vi "SwerveDrivePoseEst2_Execute.vi"(0 "Vision TImeStamp_Seconds":dbl=0.02, 3 "DiffPoseEst2Config":T3={"Wheel_Locations M"=[], "Odom X std dev M"=0.02, "Odom Y std dev M"=0.02, "Odom Heading std dev Rad"=0.01, "Vision X std dev M"=0.1, "Vision Y std dev M"=0.1, "Vision Heading std dev Rad"=0.05} {"Vision Heading std dev Rad" format="%#_13g"; "Vision Y std dev M" format="%#_13g"; "Vision X std dev M" format="%#_13g"; "Odom Heading std dev Rad" format="%#_13g"; "Odom Y std dev M" format="%#_13g"; "Odom X std dev M" format="%#_13g"; "Wheel_Locations M"."Y" format="%14.3f"; "Wheel_Locations M"."X" format="%14.3f"}, 4 "visionRobotPose":T5={"TRANSLATION"={"X"=0.0, "Y"=0.0}, "ROTATION"={"VALUE"=0.0, "COS"=1.0, "SIN"=0.0}} {"ROTATION"."SIN" format="%13.4f"; "ROTATION"."COS" format="%13.4f"; "ROTATION"."VALUE" format="%13.4f"; "TRANSLATION"."Y" format="%14.3f"; "TRANSLATION"."X" format="%14.3f"}, 5 "Game Started":bool, 6 "Add Vision Meas":bool, 7 "InitialPose":T5={"TRANSLATION"={"X"=0.0, "Y"=0.0}, "ROTATION"={"VALUE"=0.0, "COS"=1.0, "SIN"=0.0}} {"ROTATION"."SIN" format="%13.4f"; "ROTATION"."COS" format="%13.4f"; "ROTATION"."VALUE" format="%13.4f"; "TRANSLATION"."Y" format="%14.3f"; "TRANSLATION"."X" format="%14.3f"}, 8 "Pass Through Time":dbl=-1.0, 9 "Gyro Degrees":dbl, 11 "Module Positions":T1[](array[typedef]) {"Angle"."SIN" format="%13.4f"; "Angle"."COS" format="%13.4f"; "Angle"."VALUE" format="%13.4f"}) -> (1 "Error":bool, 2 "Estimated Pose":T5={"TRANSLATION"={"X"=0.0, "Y"=0.0}, "ROTATION"={"VALUE"=0.0, "COS"=1.0, "SIN"=0.0}} {"ROTATION"."SIN" format="%13.4f"; "ROTATION"."COS" format="%13.4f"; "ROTATION"."VALUE" format="%13.4f"; "TRANSLATION"."Y" format="%14.3f"; "TRANSLATION"."X" format="%14.3f"})   [LabVIEW 2019, in "Trajectory_Library.lvlib"]
uses:
  TypeDef/POSE2D.ctl
  TypeDef/TRANSLATION2D.ctl
  TypeDef/ROTATION2D.ctl
  TypeDef/SWERVE_DRIVE_POSE_EST2_CONFIG.ctl
  TypeDef/SWERVE_DRIVE_MODULE_POSITION.ctl
  Conv_Deg_Radians.vi
  Rotation2d_CreateAngle.vi
  Util_GetTime_U32.vi
  MatBuilder_Create.vi
  Util_GetTime_U64.vi
  Trajectory_Library.lvlib
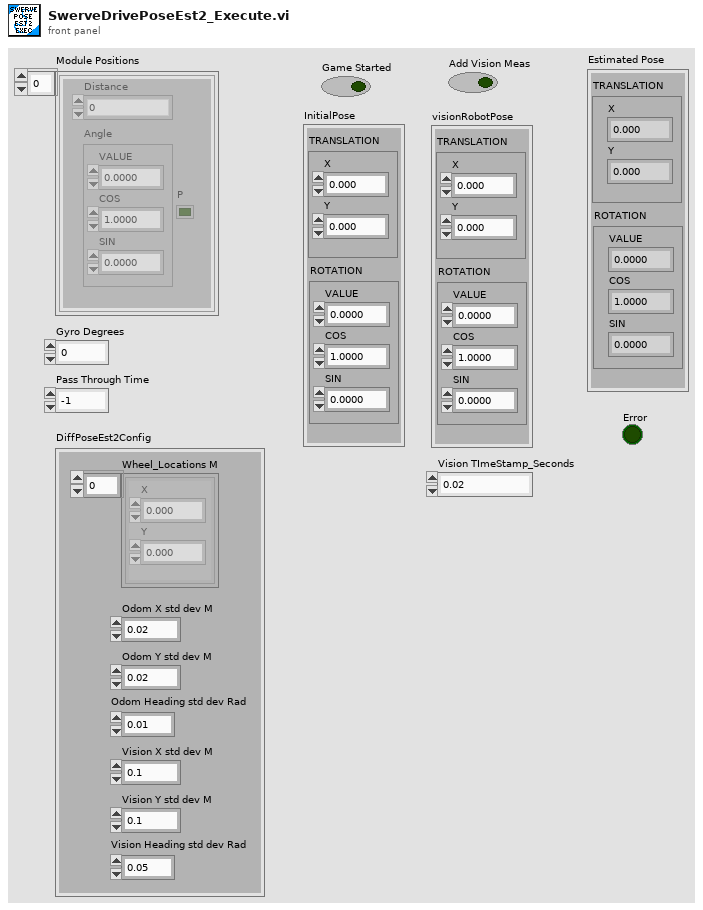
[diagram p1: front panel]
types:
  T1 = typedef "Trajectory_Library.lvlib/SWERVE_DRIVE_MODULE_POSITION.ctl" = cluster{"Distance":dbl, "Angle":T2, "P":bool}
  T2 = typedef "Trajectory_Library.lvlib/ROTATION2D.ctl" = cluster{"VALUE":dbl, "COS":dbl, "SIN":dbl}
  T3 = typedef "Trajectory_Library.lvlib/SWERVE_DRIVE_POSE_EST2_CONFIG.ctl" = cluster{"Wheel_Locations M":T4[], "Odom X std dev M":dbl, "Odom Y std dev M":dbl, "Odom Heading std dev Rad":dbl, "Vision X std dev M":dbl, "Vision Y std dev M":dbl, "Vision Heading std dev Rad":dbl}
  T4 = typedef "Trajectory_Library.lvlib/TRANSLATION2D.ctl" = cluster{"X":dbl, "Y":dbl}
  T5 = typedef "Trajectory_Library.lvlib/POSE2D.ctl" = cluster{"TRANSLATION":T4, "ROTATION":T2}
  T6 = typedef "NI_Matrix.lvlib/RealMatrix.ctl" = dbl[][]
  T7 = typedef "Trajectory_Library.lvlib/SWERVE_DRIVE_KINEMATICS.ctl" = cluster{"NumModules":i32, "InverseKinematics":T6, "ForwardKinematics":T6, "Modules":T4[], "PrevCoR":T4, "SavedModuleStates":T8[]}
  T8 = typedef "Trajectory_Library.lvlib/SWERVE_DRIVE_MODULE_STATE.ctl" = cluster{"Speed":dbl, "Angle":T2}
  T9 = typedef "Trajectory_Library.lvlib/SWERVE_DRIVE_POSE_EST2.ctl" = cluster{"M_Vision_K":T6, "m_nominal_dT":dbl, "m_PrevTime_Sec":dbl, "Pose_Buffer":T10, "Swerve_Drive_Kinematics":T7, "Swerve_Drive_Odom":T11, "M_Q":T6, "NumModules":i32}
  T10 = typedef "Trajectory_Library.lvlib/TIME_INTERPOLATABLE_VARIANT.ctl" = cluster{"TimeStamps":dbl[], "DataArray":variant[], "Min_TimeStamp":dbl, "Max_TimeStamp":dbl, "ItemCount":i32, "MaxBufferTime":dbl}
  T11 = typedef "Trajectory_Library.lvlib/SWERVE_DRIVE_ODOMETRY.ctl" = cluster{"POSE":T5, "GyroOffset":T2, "PreviousAngle":T2, "PrevModulePositions":T1[], "NumModules":i32}
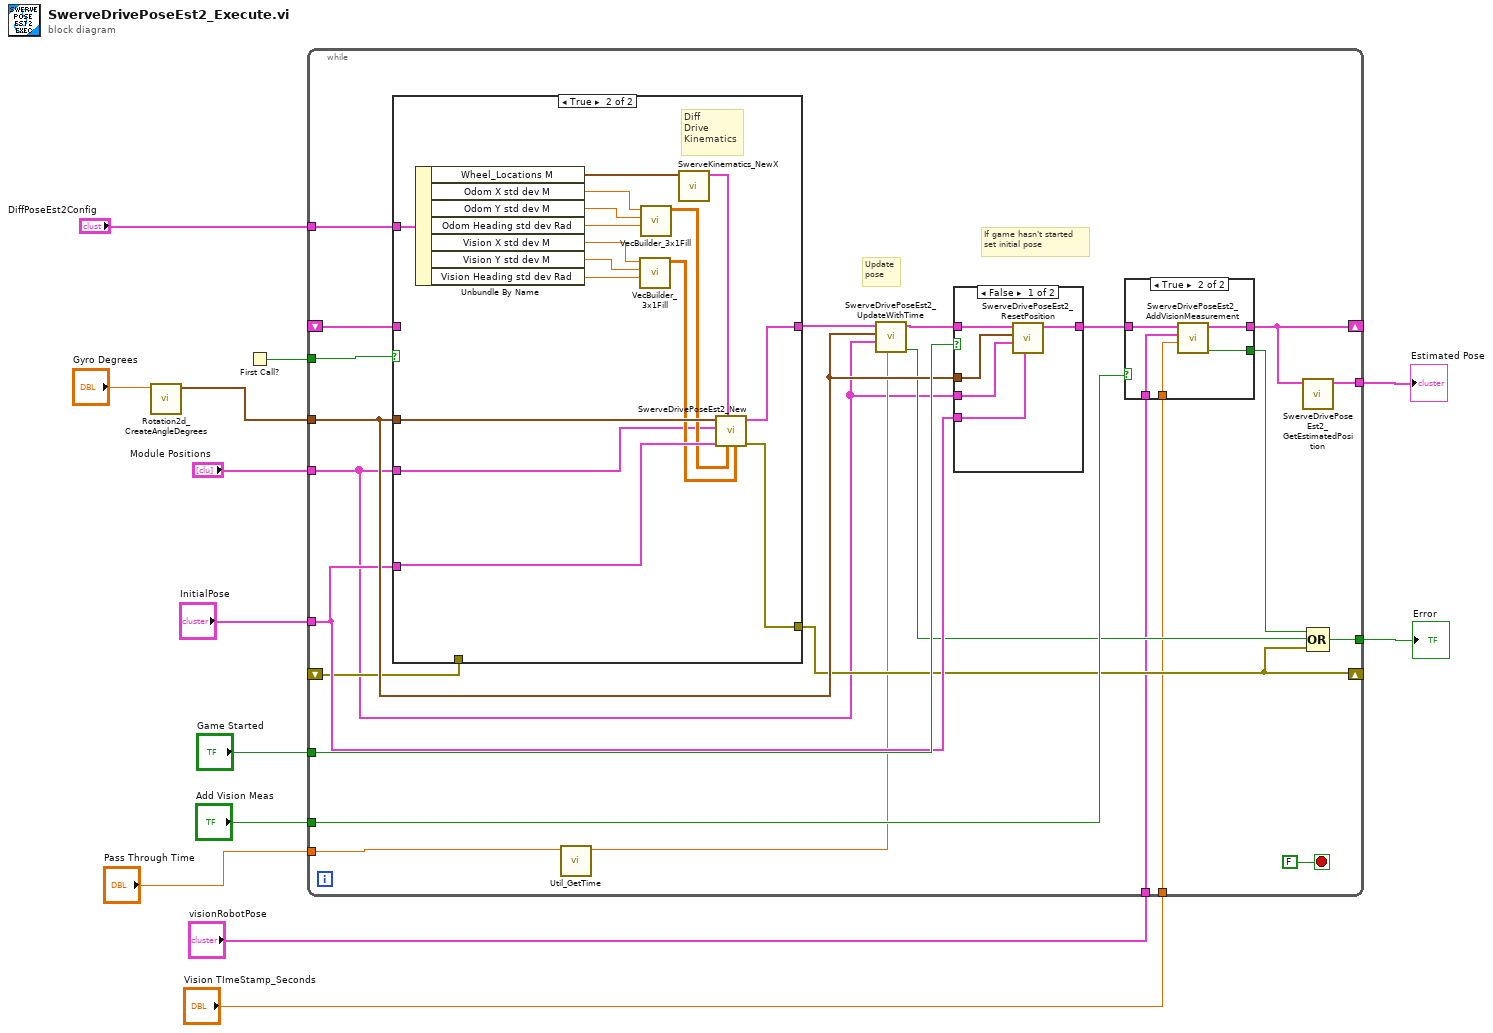
[diagram p0: block diagram]
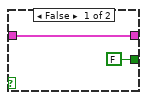
[diagram p3: hidden frame]
diagram:
  n1 = call "Rotation2d_CreateAngleDegrees.vi"("Angle_Degrees"="Gyro Degrees") -> ("ROTATION"=w4:T2)  [unwired: 10 in]
  n2 = First Call?() -> (First Call?: T/F=w13:bool)
  n3 = while {
    tunnel: w13 -> [w35]
    tunnel: w4 -> [w31]
    tunnel: "InitialPose" -> [w30]
    tunnel: "Game Started" -> [w32]
    shift-right: [w23] -> _
    shift-left: _ -> [w28]
    tunnel: "Add Vision Meas" -> [w27]
    shift-right: [w24] -> _
    shift-left: _ -> [w18]
    tunnel: [w22] -> w9
    tunnel: [w21] -> w8
    tunnel: "visionRobotPose" -> [w20]
    tunnel: "Vision TImeStamp_Seconds" -> [w19]
    tunnel: "Pass Through Time" -> [w16]
    tunnel: "DiffPoseEst2Config" -> [w15]
    tunnel: "Module Positions" -> [w14]
    stop <- FALSE stop-if-true
    # "If game hasn't started\nset initial pose"
    # "Update\npose"
    n4 = case shown="True" w35 {
      tunnel: w31 -> [_ w66]
      tunnel: w30 -> [_ w65]
      tunnel: [w50 w64] -> w24
      tunnel: [w51 w63] -> w34
      tunnel: w28 -> [w51 _]
      tunnel: w18 -> [w50 _]
      tunnel: w15 -> [_ w62]
      tunnel: w14 -> [_ w53]
      frame False {
      }
      frame True {
        # "Diff\nDrive\nKinematics"
        n5 = Unbundle By Name(w62) -> ("Wheel_Locations M"=w52:T4[], "Odom X std dev M"=w61:dbl, "Odom Y std dev M"=w60:dbl, "Odom Heading std dev Rad"=w59:dbl, "Vision X std dev M"=w58:dbl, "Vision Y std dev M"=w57:dbl, "Vision Heading std dev Rad"=w56:dbl)
        n6 = call "VecBuilder_3x1Fill.vi"("R2"=w56, "R1"=w57, "R0"=w58) -> ("output matrix"=w54:T6)  [unwired: 8 in]
        n7 = call "VecBuilder_3x1Fill.vi"("R2"=w59, "R1"=w60, "R0"=w61) -> ("output matrix"=w55:T6)  [unwired: 8 in]
        n8 = call "SwerveKinematics_NewX.vi"("Wheels"=w52) -> ("SWERVE_DRIVE_KINEMATICS"=w67:T7)  [unwired: 10 in]
        n9 = call "SwerveDrivePoseEst2_New.vi"("VisionMeasurementStdDevs"=w54, "StateStdDevs"=w55, "SWERVE_DRIVE_KINEMATICS"=w67, "InitialPose"=w65, "Module Positions"=w53, "gyroAngle"=w66) -> ("Error"=w64:errorcluster, "SwerveDrivePoseEstimate"=w63:T9)  [unwired: 4 in]
      }
    }
    n10 = call "Util_GetTime.vi"("Pass_Through_Time"=w16) -> ("FPGA_Time_Seconds"=w17:dbl)  [unwired: 8 in, 2 out]
    n11 = call "SwerveDrivePoseEst2_UpdateWithTime.vi"("CurrentTimeSeconds"=w17, "module Positions"=w14, "GyroAngle"=w31, "in SwerveDrivePoseEst2"=w34) -> ("Error"=w26:bool, "Out SwerveDrivePoseEst2"=w33:T9)  [unwired: 5 in, 1 out]
    n12 = case shown="False" w32 {
      tunnel: w33 -> [w41 w42]
      tunnel: w31 -> [w40 _]
      tunnel: w14 -> [w39 _]
      tunnel: w30 -> [w38 _]
      tunnel: [w37 w42] -> w29
      frame False {
        n13 = call "SwerveDrivePoseEst2_ResetPosition.vi"("Pose"=w38, "Module Positions"=w39, "Gyro"=w40, "in SwerveDrivePoseEst2"=w41) -> ("Out SwerveDrivePoseEst2"=w37:T9)  [unwired: 7 in]
      }
      frame True {
      }
    }
    n14 = case shown="True" w27 {
      tunnel: w29 -> [w44 w49]
      tunnel: [w44 w48] -> w23
      tunnel: [FALSE ("Error") w47] -> w25
      tunnel: w20 -> [_ w46]
      tunnel: w19 -> [_ w45]
      frame False {
      }
      frame True {
        n15 = call "SwerveDrivePoseEst2_AddVisionMeasurement.vi"("TImeStamp_Seconds"=w45, "visionRobotPose"=w46, "in SwerveDrivePoseEst2"=w49) -> ("Error"=w47:bool, "Out SwerveDrivePoseEst2"=w48:T9)  [unwired: 7 in]
      }
    }
    n16 = call "SwerveDrivePoseEst2_GetEstimatedPosition.vi"("in SwerveDrivePoseEstimate"=w23) -> ("Estimated Pose"=w22:T5)  [unwired: 10 in]
    n17 = Compound Arithmetic op=OR(w25, w26, w24) -> (w21:bool)
  }
  "Estimated Pose" <- w9
  "Error" <- w8
